vi "Write Image Receiver.vi"(8 "error in (no error)":errorcluster, 10 "Actor Framework:Message Enqueuer":refnum<class "Message Enqueuer.lvclass">, 11 "IMAQdx Actor in":refnum<class "Camera Actor.lvclass">) -> (0 "error out":errorcluster, 3 "IMAQdx Actor out":refnum<class "Camera Actor.lvclass">)   [LabVIEW 2014, in "Camera Actor.lvlib" / "Camera Actor.lvclass"]
uses:
  Camera Actor.lvclass
  <vilib>/ActorFramework/Message Enqueuer/Message Enqueuer.lvclass
  Camera Actor.lvclass/Camera Actor.ctl
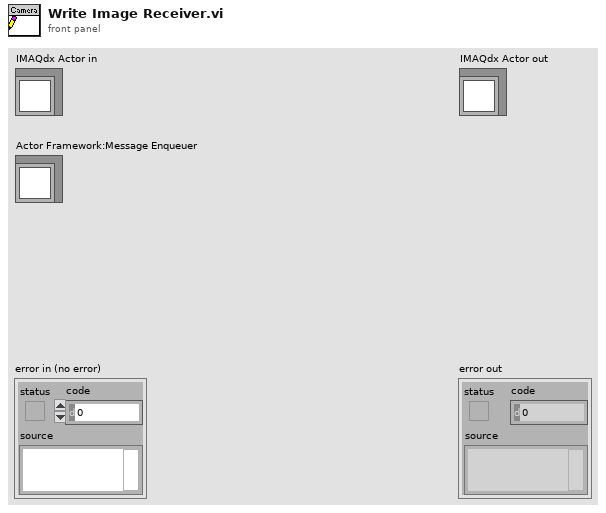
[diagram p1: front panel]
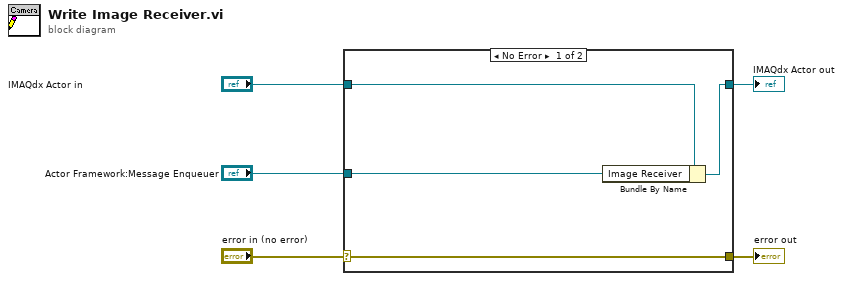
[diagram p0: block diagram]
diagram:
  n1 = case shown="No Error" "error in (no error)" {
    selector: "error in (no error)" -> [w9 w10]
    tunnel: [w9 w10] -> w4
    tunnel: [w7 w11] -> w2
    tunnel: "IMAQdx Actor in" -> [w8 w11]
    tunnel: "Actor Framework:Message Enqueuer" -> [w6 _]
    frame No Error {
      n2 = Bundle By Name(cluster=w8, "Image Receiver"=w6) -> (w7:refnum<class "Camera Actor.lvclass">)
    }
    frame Error {
    }
  }
  "error out" <- w4
  "IMAQdx Actor out" <- w2
